vi "Acquire Multi Echo .vi"(0 "VISA resource name":refnum<visa-resource-name>, 1 "Cluster Count (1)":dbl=1.0, 5 "Start Point (-120°)":dbl=-120.0, 7 "Mode (Multiecho Distance Measurement)":T1(ring), 9 "End Point (120°)":dbl=120.0, 11 "error in (no error)":errorcluster) -> (4 "VISA resource name out":refnum<visa-resource-name>, 6 "Magnitude Array":i32[][](array[numeric]), 8 "Reflected Intensity Array":i32[][](array[numeric]), 10 "Direction":dbl[](array[numeric]), 15 "error out":errorcluster)   [LabVIEW 2014, in "Hokuyo URG Series.lvlib"]
doc: "This VI takes three parameters (start point, end point, cluster count) and returns two arrays which describe the magnitude and angle at which the data was acquired. \n\nThe reference for the angles (in the Direction array) is the center of the device which is 0° with positive angles to the left of center and negative angles to the right.\n\nThe URG-04LX can take measurements in the range of -120° to 120° and has an \"operating range\" of -135° to 135°. \n\nCluster Count refers to the number of measurements which are clustered together. \n<b>Ex:</b>If the cluster count is 3 then the smallest of three measurements is returned.\n\nThe Magnitude array is associated with the Direction array. \n<b>Ex:</b> If the information for the first measurement is desired, then the 0th index of each array is accessed and returns the magnitude and direction of the first measurement.\n\nIf checksums are being used and the checksum fails, the data returned in the magnitude array will default to -1."
uses:
  Hokuyo URG Series.lvlib
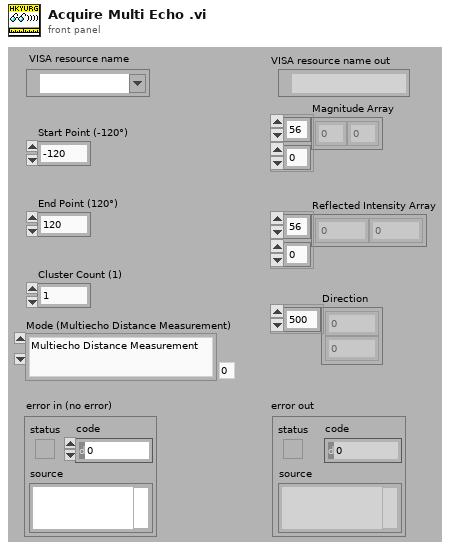
[diagram p1: front panel]
types:
  T1 = enum16{"Multiecho Distance Measurement", "Multiecho Distance and Reflected Intensity Measurement"}
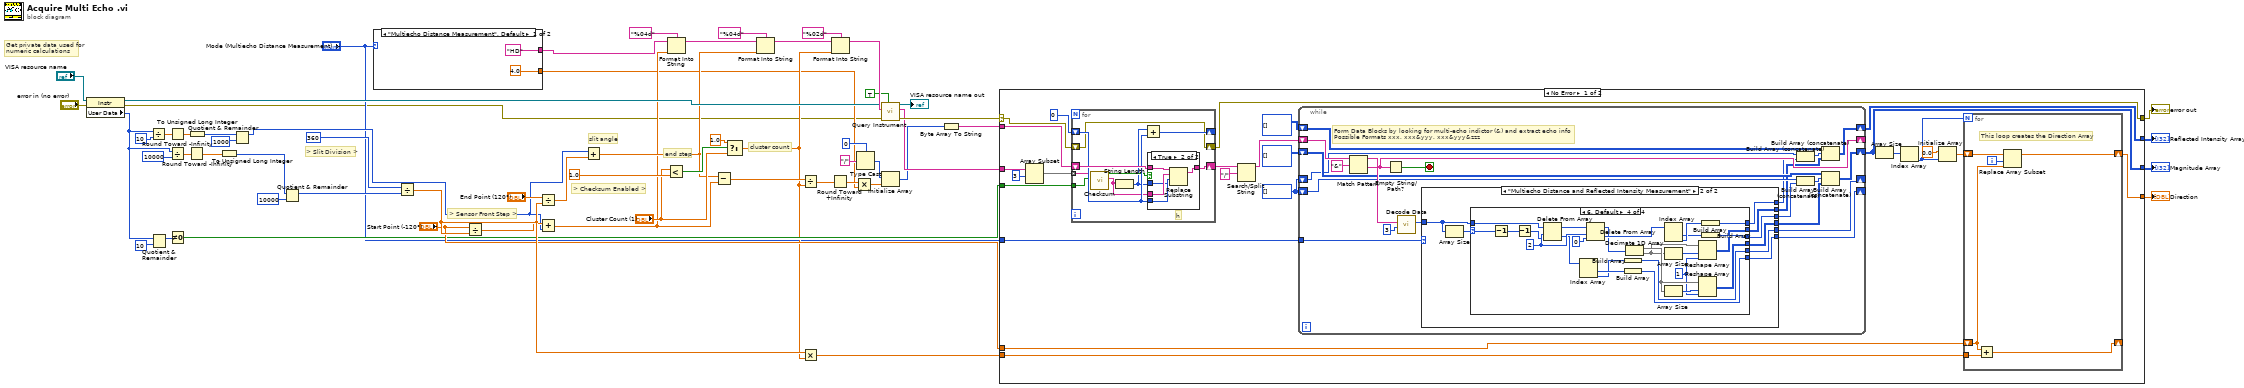
[diagram p0: block diagram]
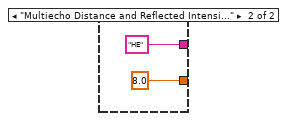
[diagram p2: hidden frame]
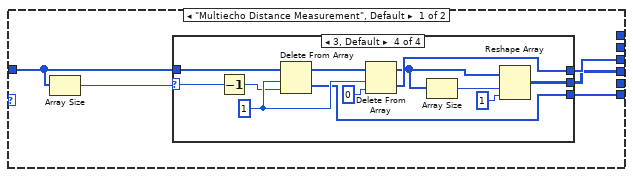
[diagram p3: hidden frame]
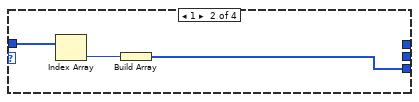
[diagram p5: hidden frame]
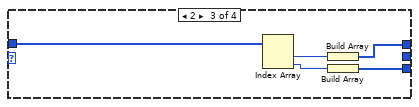
[diagram p6: hidden frame]
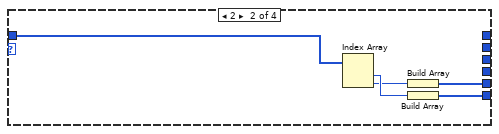
[diagram p8: hidden frame]
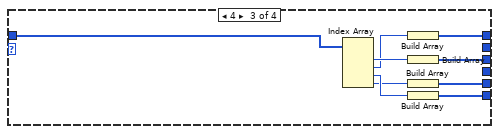
[diagram p9: hidden frame]
diagram:
  # "> Checksum Enabled >"
  # "Get private data used for numeric calculations"
  # "> Slit Division >"
  # "> Sensor Front Step >"
  # "cluster count"
  # "end step"
  # "slit angle"
  n1 = property class="Instr"(reference="VISA resource name", error in="error in (no error)") -> (reference out=w27:refnum<visa-resource-name>, error out=w1:errorcluster, "User Data"=w20:u32)
  n2 = Divide(x=w20, y=u32 10) -> (x/y=w40:dbl)
  n3 = Quotient & Remainder(x=w20, y=u32 10) -> (x-y*floor(x/y)=w21:u32)  [unwired: 1 out]
  n4 = Round Toward -Infinity(1:w40) -> (0:w37:dbl)
  n5 = Divide(x=w20, y=u32 10000) -> (x/y=w35:dbl)
  n6 = Not Equal To 0?(x=w21) -> (x != 0?=w19:bool)
  n7 = To Unsigned Long Integer(number=w37) -> (unsigned 32bit integer=w39:u32)
  n8 = Round Toward -Infinity(1:w35) -> (0:w34:dbl)
  n9 = To Unsigned Long Integer(number=w34) -> (unsigned 32bit integer=w33:u32)
  n10 = Quotient & Remainder(x=w39, y=u32 1000) -> (x-y*floor(x/y)=w38:u32)  [unwired: 1 out]
  n11 = Quotient & Remainder(x=w33, y=u32 10000) -> (x-y*floor(x/y)=w31:u32)  [unwired: 1 out]
  n12 = case shown="\"Multiecho Distance Measurement\", Default" "Mode (Multiecho Distance Measurement)" {
    tunnel: ["HD" ("initial string") "HE" ("initial string")] -> w5
    tunnel: [4.0 ("y") 8.0 ("y")] -> w4
    frame "Multiecho Distance Measurement", Default {
    }
    frame "Multiecho Distance and Reflected Intensity Measurement" {
    }
  }
  n13 = Divide(x=u32 360 ("y"), y=w31) -> (x/y=w46:dbl)
  n14 = Divide(x="Start Point (-120°)", y=w46) -> (x/y=w44:dbl)
  n15 = Divide(x="End Point (120°)", y=w46) -> (x/y=w42:dbl)
  n16 = Add(x=w44, y=w38) -> (x+y=w8:dbl)
  n17 = Add(x=w38, y=w42) -> (x+y=w11:dbl)
  n18 = Less?(x="Cluster Count (1)", y=1.0) -> (x < y?=w50:bool)
  n19 = Format Into String(format string="%04d", initial string=w5, w8) -> (resulting string=w56:string)  [unwired: 1 in, 1 out]
  n20 = Subtract(x=w11, y=w8) -> (x-y=w13:dbl)
  n21 = Select(t=1.0, s=w50, f="Cluster Count (1)") -> (s? t:f=w7:dbl)
  n22 = Format Into String(format string="%04d", initial string=w56, w11) -> (resulting string=w54:string)  [unwired: 1 in, 1 out]
  n23 = Divide(x=w13, y=w7) -> (x/y=w12:dbl)
  n24 = Multiply(x=w46, y=w7) -> (x*y=w52:dbl)
  n25 = Round Toward +Infinity(x=w12) -> (ceil(x): smallest int >= x=w10:dbl)
  n26 = Format Into String(format string="%02d", initial string=w54, w7) -> (resulting string=w53:string)  [unwired: 1 in, 1 out]
  n27 = Multiply(x=w10, y=w4) -> (x*y=w15:dbl)
  n28 = Type Cast(type=u8 0, x="/") -> (*(type *) &x=w18:u8)
  n29 = call "Query Instrument.vi"("Error Query (Enabled)"=TRUE, "error in"=w1, "Command"=w53, "VISA Resource Name"=w27) -> ("error out"=w24:errorcluster, "Response Strings"=w23:string[], "VISA Resource Name Out"=→"VISA resource name out":refnum<visa-resource-name>)  [unwired: 5 in]
  n30 = Initialize Array(w18, w15) -> (w14:u8[])
  n31 = Byte Array To String(unsigned byte array=w14) -> (string=w9:string)
  n32 = case shown="No Error" w24 {
    selector: w24 -> [w78 w205]
    tunnel: [w77 w205] -> w59
    tunnel: "Start Point (-120°)" -> [w88 _]
    tunnel: w52 -> [w87 _]
    tunnel: [w86 _] -> w60
    tunnel: w23 -> [w82 _]
    tunnel: w19 -> [w80 _]
    tunnel: w9 -> [w76 _]
    tunnel: [w70 _] -> w6
    tunnel: "Mode (Multiecho Distance Measurement)" -> [w69 _]
    tunnel: [w65 _] -> w2
    frame No Error {
      w66 = i32[] []
      n33 = Array Subset(array=w82, index=3 ("y")) -> (w81:string[])  [unwired: 1 in]
      n34 = for {
        shift-right: [w184] -> w77
        shift-left: w78 -> [w184]
        shift-right: [w192] -> w73
        shift-left: w76 -> [w191]
        shift-right: [w189] -> _
        shift-left: 0 -> [w190]
        tunnel: w80 -> [w187]
        tunnel: w81 -> [w183] mode=indexing
        # "h"
        n35 = call "Checksum.vi"("Checksum (Off)"=w187, "Input"=w183) -> ("Data Buffer"=w186:string, "Checksum Pass?"=w188:bool)  [unwired: 8 out]
        n36 = String Length(string=w186) -> (length=w185:i32)
        n37 = Add(x=w185, y=w190) -> (x+y=w189:i32)
        n38 = case shown="True" w188 {
          tunnel: [w193 w194] -> w192
          tunnel: w191 -> [w193 w198]
          tunnel: w186 -> [_ w197]
          tunnel: w190 -> [_ w196]
          tunnel: w185 -> [_ w195]
          frame False {
          }
          frame True {
            n39 = Replace Substring(2:w195, 3:w196, 4:w197, 5:w198) -> (1:w194:string)  [unwired: 1 out]
          }
        }
      }
      n40 = Search/Split String(string=w73, search string/char (-)="/") -> (substring before match=w71:string)  [unwired: 1 in, 2 out]
      n41 = while {
        shift-right: [w102] -> _
        shift-left: w71 -> [w110]
        shift-right: [w104] -> _
        shift-left: w66 -> [w106]
        shift-right: [w103] -> w70
        shift-left: i32[][] [] -> [w99]
        tunnel: w69 -> [w96]
        shift-right: [w92] -> w65
        shift-left: i32[][] [] -> [w95]
        shift-right: [w91] -> _
        shift-left: w66 -> [w94]
        stop <- w101 stop-if-true
        # "Form Data Blocks by looking for multi-echo indictor (&) and extract echo info \nPossible Formats xxx, xxx&yyy, xxx&yyy&zzz"
        n42 = Match Pattern(string=w110, regular expression="&") -> (before substring=w109:string, after substring=w102:string)  [unwired: 1 in, 2 out]
        n43 = Empty String/Path?(string/path=w102) -> (empty?=w101:bool)
        n44 = call "Decode Data.vi"("n character encoding"=u32 3, "Input Buffer"=w109) -> ("Decoded Measurements"=w107:i32[])  [unwired: 3 in, 6 out]
        n45 = case shown="\"Multiecho Distance and Reflected Intensity Measurement\"" w96 {
          tunnel: w107 -> [w114 w142]
          tunnel: [w113 w141] -> w105
          tunnel: [w112 w140] -> w104
          tunnel: [w111 w139] -> w97
          tunnel: [_ w138] -> w91
          tunnel: [_ w137] -> w90
          tunnel: [_ w136] -> w89
          frame "Multiecho Distance Measurement", Default {
            n46 = Array Size(array=w114) -> (size(s)=w115:i32)
            n47 = case shown="3, Default" w115 {
              selector: w115 -> [_ _ _ w135]
              tunnel: w114 -> [_ w118 w123 w129]
              tunnel: [_ _ w121 w133] -> w113
              tunnel: [_ w116 w119 w130] -> w112
              tunnel: [_ _ _ w126] -> w111
              frame 0 {
              }
              frame 1 {
                n48 = Index Array(array=w118) -> (element=w117:i32)  [unwired: 1 in]
                n49 = Build Array(w117) -> (w116:i32[])
              }
              frame 2 {
                n50 = Index Array(array=w123) -> (element #1=w122:i32, element #2=w120:i32)  [unwired: 2 in]
                n51 = Build Array(w122) -> (w121:i32[])
                n52 = Build Array(w120) -> (w119:i32[])
              }
              frame 3, Default {
                w132 = 1 ("length")
                n53 = Decrement(x=w135) -> (x-1=w131:i32)
                n54 = Delete From Array(array=w129, length=w132, index=w131) -> (deleted portion=w130:i32[], array with subset deleted=w128:i32[])
                n55 = Delete From Array(array=w128, length=w132, index=0) -> (deleted portion=w133:i32[], array with subset deleted=w127:i32[])
                n56 = Array Size(array=w127) -> (size(s)=w125:i32)
                n57 = Reshape Array(w127, w125, 1 ("dimension size")) -> (w126:i32[][])
              }
            }
          }
          frame "Multiecho Distance and Reflected Intensity Measurement" {
            n58 = Array Size(array=w142) -> (size(s)=w143:i32)
            n59 = case shown="6, Default" w143 {
              selector: w143 -> [_ _ _ w182]
              tunnel: w142 -> [_ w148 w157 w179]
              tunnel: [_ _ w155 w165] -> w141
              tunnel: [_ w146 w154 w170] -> w140
              tunnel: [_ _ _ w177] -> w139
              tunnel: [_ w144 w149 w169] -> w138
              tunnel: [_ _ w151 w164] -> w137
              tunnel: [_ _ _ w158] -> w136
              frame 0 {
              }
              frame 2 {
                n60 = Index Array(array=w148) -> (element #1=w147:i32, element #2=w145:i32)  [unwired: 2 in]
                n61 = Build Array(w145) -> (w144:i32[])
                n62 = Build Array(w147) -> (w146:i32[])
              }
              frame 4 {
                n63 = Index Array(array=w157) -> (element #1=w156:i32, element #2=w152:i32, element #3=w153:i32, element #4=w150:i32)  [unwired: 4 in]
                n64 = Build Array(w152) -> (w151:i32[])
                n65 = Build Array(w156) -> (w155:i32[])
                n66 = Build Array(w150) -> (w149:i32[])
                n67 = Build Array(w153) -> (w154:i32[])
              }
              frame 6, Default {
                w160 = 1 ("dimension size")
                w180 = 2 ("length")
                n68 = Decrement(x=w182) -> (x-1=w175:i32)
                n69 = Decrement(x=w175) -> (x-1=w174:i32)
                n70 = Delete From Array(array=w179, length=w180, index=w174) -> (deleted portion=w173:i32[], array with subset deleted=w178:i32[])
                n71 = Index Array(array=w173) -> (element #1=w172:i32, element #2=w171:i32)  [unwired: 2 in]
                n72 = Delete From Array(array=w178, length=w180, index=0) -> (deleted portion=w166:i32[], array with subset deleted=w163:i32[])
                n73 = Build Array(w171) -> (w169:i32[])
                n74 = Build Array(w172) -> (w170:i32[])
                n75 = Decimate 1D Array(w163) -> (w162:i32[], w159:i32[])
                n76 = Index Array(array=w166) -> (element #1=w167:i32, element #2=w168:i32)  [unwired: 2 in]
                n77 = Array Size(array=w159) -> (size(s)=w161:i32)
                n78 = Array Size(array=w162) -> (size(s)=w176:i32)
                n79 = Reshape Array(w159, w161, w160) -> (w158:i32[][])
                n80 = Reshape Array(w162, w176, w160) -> (w177:i32[][])
                n81 = Build Array(w168) -> (w164:i32[])
                n82 = Build Array(w167) -> (w165:i32[])
              }
            }
          }
        }
        n83 = Build Array (concatenate)(w94, w90) -> (w93:i32[])
        n84 = Build Array (concatenate)(w106, w105) -> (w98:i32[])
        n85 = Build Array (concatenate)(w95, w93, w89) -> (w92:i32[][])
        n86 = Build Array (concatenate)(w99, w98, w97) -> (w103:i32[][])
      }
      n87 = Array Size(array=w70) -> (size(s)=w75:i32[])
      n88 = Index Array(array=w75) -> (element=w68:i32)  [unwired: 1 in]
      n89 = Initialize Array(0.0 ("element"), w68) -> (w84:dbl[])
      n90 = for {
        N: w68 -> [_]
        shift-right: [w203] -> _
        shift-left: w88 -> [w200]
        tunnel: w87 -> [w204]
        shift-right: [w201] -> w86
        shift-left: w84 -> [w202]
        i -> [w199]
        # "This loop creates the Direction Array"
        n91 = Add(x=w200, y=w204) -> (x+y=w203:dbl)
        n92 = Replace Array Subset(array=w202, new element=w200, index=w199) -> (w201:dbl[])
      }
    }
    frame Error {
    }
  }
  "Direction" <- w60
  "error out" <- w59
  "Magnitude Array" <- w6
  "Reflected Intensity Array" <- w2
